vi "Configure.vi"(8 "error in (no error)":errorcluster caption="错误输入（无错误）", 11 "Simulation DMM 输入":refnum<class "Simulation DMM.lvclass">) -> (0 "error out":errorcluster caption="错误输出", 3 "Simulation DMM 输出":refnum<class "Simulation DMM.lvclass">)   [LabVIEW 2020, in "Simulation DMM.lvlib" / "Simulation DMM.lvclass"]
uses:
  Simulation DMM.lvclass
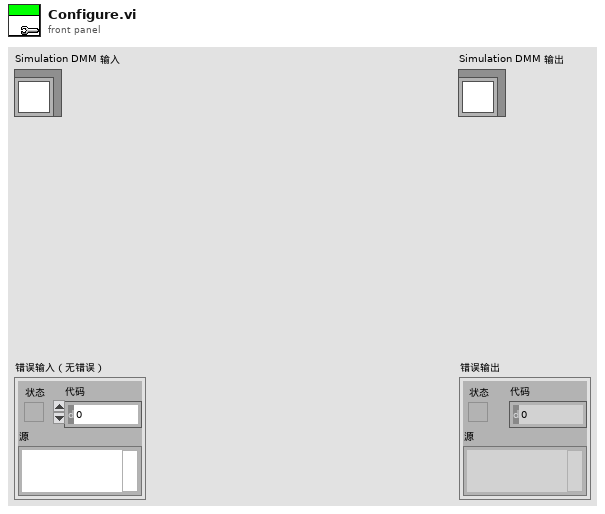
[diagram p1: front panel]
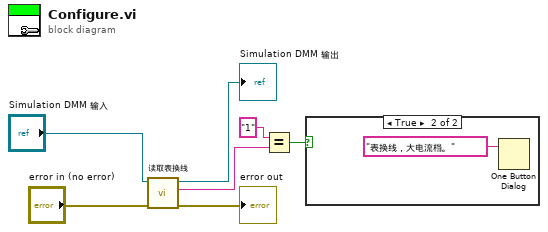
[diagram p0: block diagram]
diagram:
  n1 = call "读取表换线.vi"("error in (no error)"="error in (no error)", "数字多用表接口输入"="Simulation DMM 输入") -> ("error out"=→"error out":errorcluster, "表换线"=w4:string, "数字多用表接口输出"=→"Simulation DMM 输出":refnum<class "Simulation DMM.lvclass">)  [unwired: 7 in]
  n2 = Equal?(x="1" ("y"), y=w4) -> (x = y?=w3:bool)
  n3 = case shown="True" w3 {
    frame False {
    }
    frame True {
      n4 = One Button Dialog(message="表换线，大电流档。" ("消息")) -> ()  [unwired: 1 in, 1 out]
    }
  }
